vi "dU Puffer.vi"(8 "error in":errorcluster, 10 "Bemenõ adatok":dbl[][](array[numeric]) format="%0.2f", 11 "Analog data":T1) -> (0 "error out":errorcluster, 3 "Analog data out":T1)   [LabVIEW 2014]
uses:
  Analog data.ctl
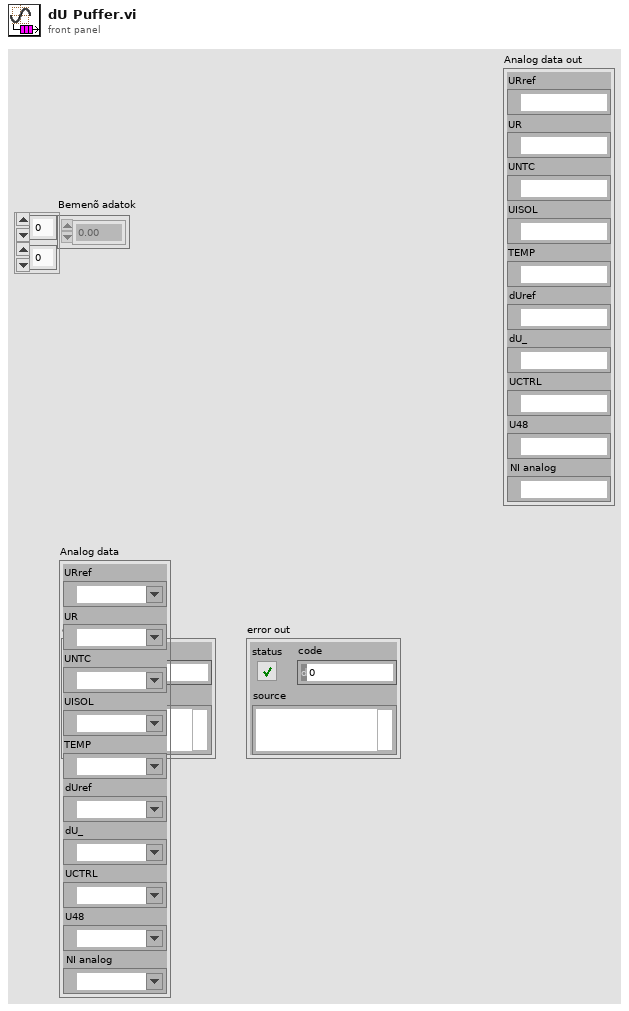
[diagram p1: front panel]
types:
  T1 = typedef "Analog data.ctl" = cluster{"URref":refnum<k21>, "UR":refnum<k21>, "UNTC":refnum<k21>, "UISOL":refnum<k21>, "TEMP":refnum<k21>, "dUref":refnum<k21>, "dU_":refnum<k21>, "UCTRL":refnum<k21>, "U48":refnum<k21>, "NI analog":refnum<k21>}
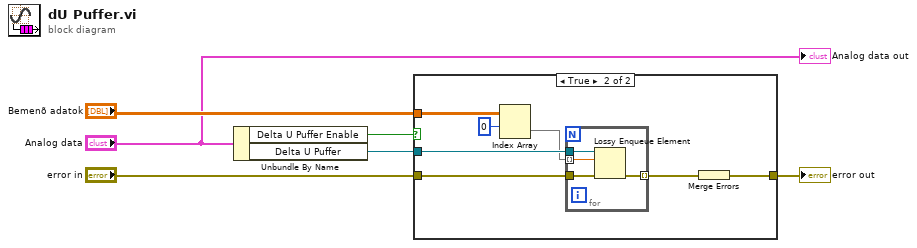
[diagram p0: block diagram]
diagram:
  n1 = Unbundle By Name("Analog data") -> ("Delta U Puffer Enable"=w3:bool, "Delta U Puffer"=w4:refnum<queue>)
  n2 = case shown="True" w3 {
    tunnel: "Bemenõ adatok" -> [_ w14]
    tunnel: w4 -> [_ w12]
    tunnel: "error in" -> [w7 w10]
    tunnel: [w7 w8] -> w1
    frame False {
    }
    frame True {
      n3 = Index Array(array=w14, index (row)=0) -> (element=w11:dbl[])  [unwired: 1 in]
      n4 = for {
        tunnel: w12 -> [w18]
        tunnel: w11 -> [w17] mode=indexing
        tunnel: w10 -> [w16]
        tunnel: [w15] -> w9 mode=indexing
        n5 = Lossy Enqueue Element(queue=w18, element=w17, error in (no error)=w16) -> (error out=w15:errorcluster)  [unwired: 3 out]
      }
      n6 = Merge Errors(w9) -> (w8:errorcluster)
    }
  }
  "error out" <- w1
  "Analog data out" <- "Analog data"
